vi "Init Shared Vars.vi"(1 "error in":errorcluster) -> (0 "error out":errorcluster)   [LabVIEW 2012]
uses:
  testing/ui_override_opts.ctl
  <vilib>/Analysis/7linalg.llb/Create Special Real Matrix.vi
  testing/ui_globals.vi
  <vilib>/Analysis/NI_AALPro.lvlib
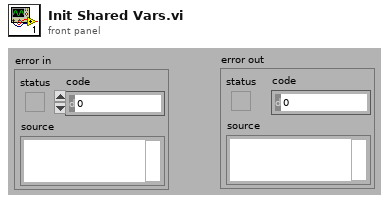
[diagram p1: front panel]
types:
  T1 = typedef "ui_override_opts.ctl" = cluster{"Triggering":bool, "Parameters":bool, "Stimulus":bool, "Calibration":bool, "Modes":bool}
  T2 = typedef "NI_Matrix.lvlib/RealMatrix.ctl" = dbl[][]
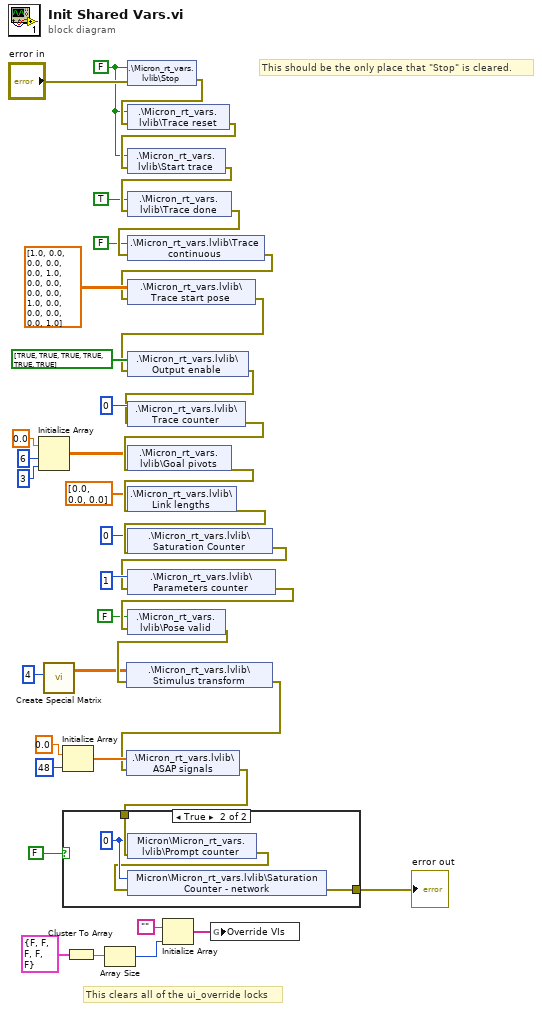
[diagram p0: block diagram]
diagram:
  w38 = FALSE
  # "This clears all of the ui_override locks"
  # "This should be the only place that \"Stop\" is cleared."
  n1 = Initialize Array(sgl 0.0 ("Numeric"), 6 ("dimension size"), 3 ("dimension size")) -> (w23:sgl[][])
  n2 = call-poly <vilib>:"Create Special Matrix.vi"("matrix size"=4) -> ("Special Matrix"=w21:T2)  [unwired: 4 in, 1 out]
  n3 = Initialize Array(sgl 0.0 ("element"), 48 ("dimension size")) -> (w12:sgl[])
  n4 = Cluster To Array(cluster=T1 {"Triggering"=FALSE, "Parameters"=FALSE, "Stimulus"=FALSE, "Calibration"=FALSE, "Modes"=FALSE} ("Override")) -> (array=w16:bool[])
  n5 = Array Size(array=w16) -> (size(s)=w15:i32)
  n6 = shared-variable ".\\Micron_rt_vars.lvlib\\Stop"(w38, error in="error in") -> (error out=w40:errorcluster)
  n7 = shared-variable ".\\Micron_rt_vars.lvlib\\Trace reset"(w38, error in=w40) -> (error out=w39:errorcluster)
  n8 = shared-variable ".\\Micron_rt_vars.lvlib\\Start trace"(w38, error in=w39) -> (error out=w7:errorcluster)
  n9 = shared-variable ".\\Micron_rt_vars.lvlib\\Trace done"(TRUE ("Trace done"), error in=w7) -> (error out=w5:errorcluster)
  n10 = shared-variable ".\\Micron_rt_vars.lvlib\\Trace continuous"(FALSE ("Trace continuous"), error in=w5) -> (error out=w1:errorcluster)
  n11 = shared-variable ".\\Micron_rt_vars.lvlib\\Trace start pose"(sgl[][] [[1.0, 0.0, 0.0, 0.0], [0.0, 1.0, 0.0, 0.0], [0.0, 0.0, 1.0, 0.0], [0.0, 0.0, 0.0, 1.0]] ("Trace start pose"), error in=w1) -> (error out=w2:errorcluster)
  n12 = shared-variable ".\\Micron_rt_vars.lvlib\\Output enable"(bool[] [TRUE, TRUE, TRUE, TRUE, TRUE, TRUE] ("Output enable"), error in=w2) -> (error out=w14:errorcluster)
  n13 = shared-variable ".\\Micron_rt_vars.lvlib\\Trace counter"(u32 0 ("Trace counter"), error in=w14) -> (error out=w36:errorcluster)
  n14 = shared-variable ".\\Micron_rt_vars.lvlib\\Goal pivots"(w23, error in=w36) -> (error out=w35:errorcluster)
  n15 = shared-variable ".\\Micron_rt_vars.lvlib\\Link lengths"(sgl[] [0.0, 0.0, 0.0] ("Goal position"), error in=w35) -> (error out=w33:errorcluster)
  n16 = shared-variable ".\\Micron_rt_vars.lvlib\\Saturation Counter"(u32 0 ("Saturation Counter"), error in=w33) -> (error out=w29:errorcluster)
  n17 = shared-variable ".\\Micron_rt_vars.lvlib\\Parameters counter"(u32 1 ("Parameters counter"), error in=w29) -> (error out=w42:errorcluster)
  n18 = shared-variable ".\\Micron_rt_vars.lvlib\\Pose valid"(FALSE ("Pose valid"), error in=w42) -> (error out=w22:errorcluster)
  n19 = shared-variable ".\\Micron_rt_vars.lvlib\\Stimulus transform"(w21, error in=w22) -> (error out=w9:errorcluster)
  n20 = shared-variable ".\\Micron_rt_vars.lvlib\\ASAP signals"(w12, error in=w9) -> (error out=w8:errorcluster)
  n21 = case shown="True" FALSE {
    tunnel: w8 -> [w43 w47]
    tunnel: [w43 w44] -> w27
    frame False {
      # "Problem with net shared vars?"
    }
    frame True {
      w46 = u32 0 ("Prompt counter")
      n22 = shared-variable "Micron\\Micron_rt_vars.lvlib\\Prompt counter"(w46, error in=w47) -> (error out=w45:errorcluster)
      n23 = shared-variable "Micron\\Micron_rt_vars.lvlib\\Saturation Counter - network"(w46, error in=w45) -> (error out=w44:errorcluster)
    }
  }
  "error out" <- w27
  n24 = Initialize Array("", w15) -> (w19:string[])
  n25 = global write "ui_globals.vi" "Override VIs"(w19) -> ()
